vi "Main.vi"() -> ()   [LabVIEW 2019]
uses:
  Control Timer.ctl
  <vilib>/vision/Image Controls.llb/IMAQ Image.ctl
  <vilib>/Utility/file.llb/Read Delimited Spreadsheet (string).vi
panel:
  out "Camera Feed":T1(plugin-control)
  in  "Empty Spot":bool
  in  "Spot Number":i8(knob)=1 scale=1.0..6.0
  in  "SnapPhoto":bool
  in  "Tab Control":T2(tab)
  out "Parking Spot #6":T3
  out "Time of Arrival 6":timestamp
  out "Ticket Expiration Time 6":timestamp
  out "Ticket Validation\n          Status 6":bool
  out "Ticket Length\n(Seconds) 6":dbl
  out "Time left\n(Seconds) 6":dbl
  out "Parking Spot #5":T3
  out "Time left\n(Seconds) 5":dbl
  out "Ticket Validation\n          Status 5":bool
  out "Time of Arrival 5":timestamp
  out "Ticket Expiration Time 5":timestamp
  out "Ticket Length\n(Seconds) 5":dbl
  out "Parking Spot #4":T3
  out "Time left\n(Seconds) 4":dbl
  out "Time of Arrival 4":timestamp
  out "Ticket Validation\n          Status 4":bool
  out "Ticket Expiration Time 4":timestamp
  out "Ticket Length\n(Seconds) 4":dbl
  out "Parking Spot #3 (Reserved for Handicapped people)":T3
  out "Ticket Validation\n          Status 3":bool
  out "Ticket Expiration Time 3":timestamp
  out "Time of Arrival 3":timestamp
  out "Ticket Length\n(Seconds) 3":dbl
  out "Time left\n(Seconds) 3":dbl
  out "Parking Spot #2":T3
  out "Time left\n(Seconds) 2":dbl
  out "Time of Arrival 2":timestamp
  out "Ticket Validation\n          Status 2":bool
  out "Ticket Expiration Time 2":timestamp
  out "Ticket Length\n(Seconds) 2":dbl
  out "Ticket Expiration Time":timestamp
  out "Time of Arrival":timestamp
  out "Ticket Validation\n          Status":bool
  out "Parking Spot #1":T3
  out "Time left\n(Seconds)":dbl
  out "Ticket Length\n(Seconds)":dbl
  in  "UseCamera":bool
  out "Error Terminal Out":errorcluster
  in  "Licence Database filepath":path=path "C:/Users/nedel/Desktop/PSR 'Veljko' Mk.Ia/Files/Databases/LicenceDatabase.csv"
  out "error out 6":errorcluster
  out "error out 5":errorcluster
  out "error out":errorcluster
  out "error out 4":errorcluster
  out "error out 2":errorcluster
  out "error out 3":errorcluster
  in  "Ticket Database filepath":path=path "C:/Users/nedel/Desktop/PSR 'Veljko' Mk.Ia/Files/Databases/TicketDatabase.csv"
  in  "Criminal record database":path=path "C:/Users/nedel/Desktop/PSR 'Veljko' Mk.Ia/Files/Databases/CriminalRecordsDatabase.csv"
  in  "Python program filepath":path=path "C:/Users/nedel/Desktop/PSR 'Veljko' Mk.Ia/Python/gopro.py"
  in  "Handicapped Right Database":path=path "C:/Users/nedel/Desktop/PSR 'Veljko' Mk.Ia/Files/Databases/HandicappedRightDatabase.csv"
  in  "ImageFilepath":path=path "C:/Users/nedel/Desktop/PSR 'Veljko' Mk.Ia/Python/gopro.py"
  in  "stop":bool
  # "SCADA controls"
  # "Image acquisition might take some time\ndue to hardware limitations\n(Approximately 10 seconds)"
  # "!"
  # "6"
  # "5"
  # "4"
  # "3"
  # "2"
  # "1"
  # "UseFile"
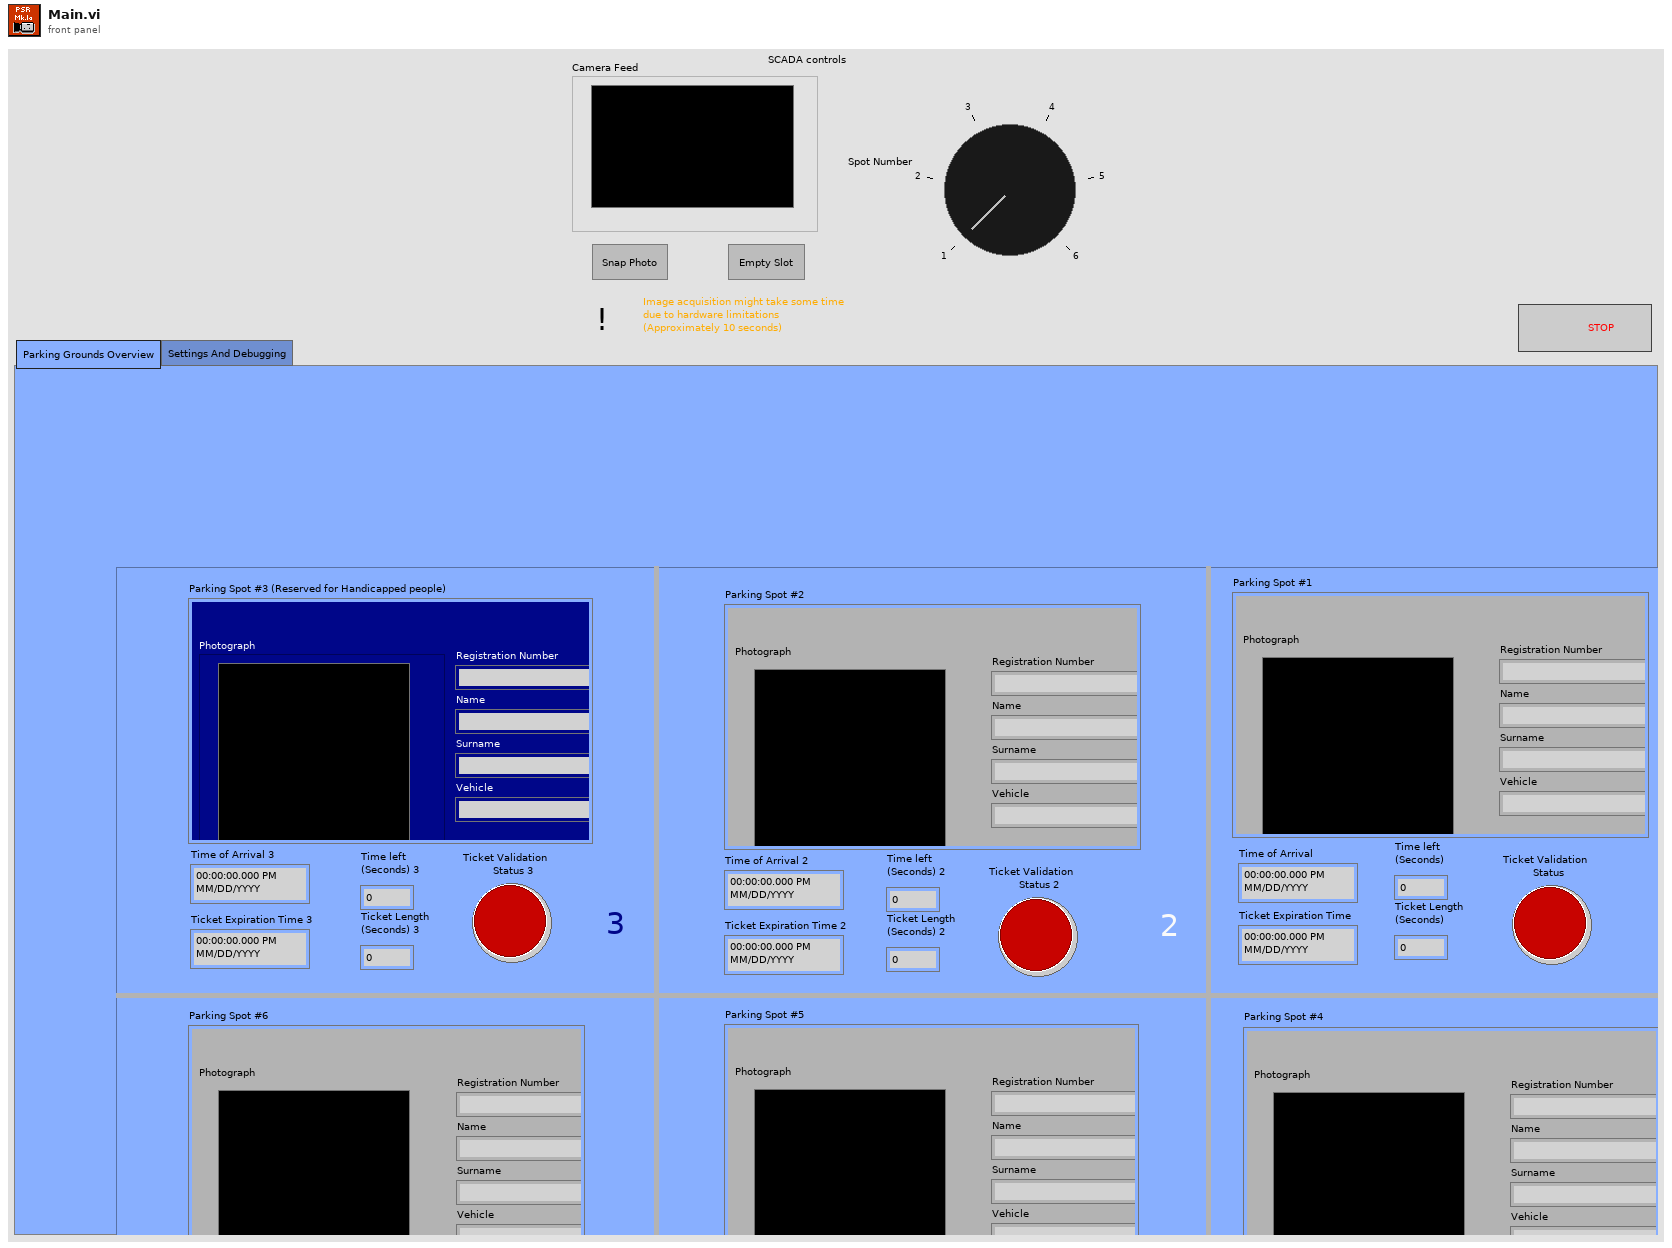
[diagram p1: front panel]
types:
  T1 = typedef "IMAQ Image.ctl" = refnum<image>
  T2 = enum32{"Parking Grounds Overview", "Settings And Debugging"}
  T3 = cluster{"Registration Number":string, "Name":string, "Surname":string, "Vehicle":string, "Photograph":T1}
  T4 = cluster{"Registration Number":string, "Name":string, "Surname":string, "Place":string, "Photograph":T1}
  T5 = typedef "Control Timer.ctl" = enum16{"Timecheck", "Reset"}
  T6 = typedef "Image Type" = u32
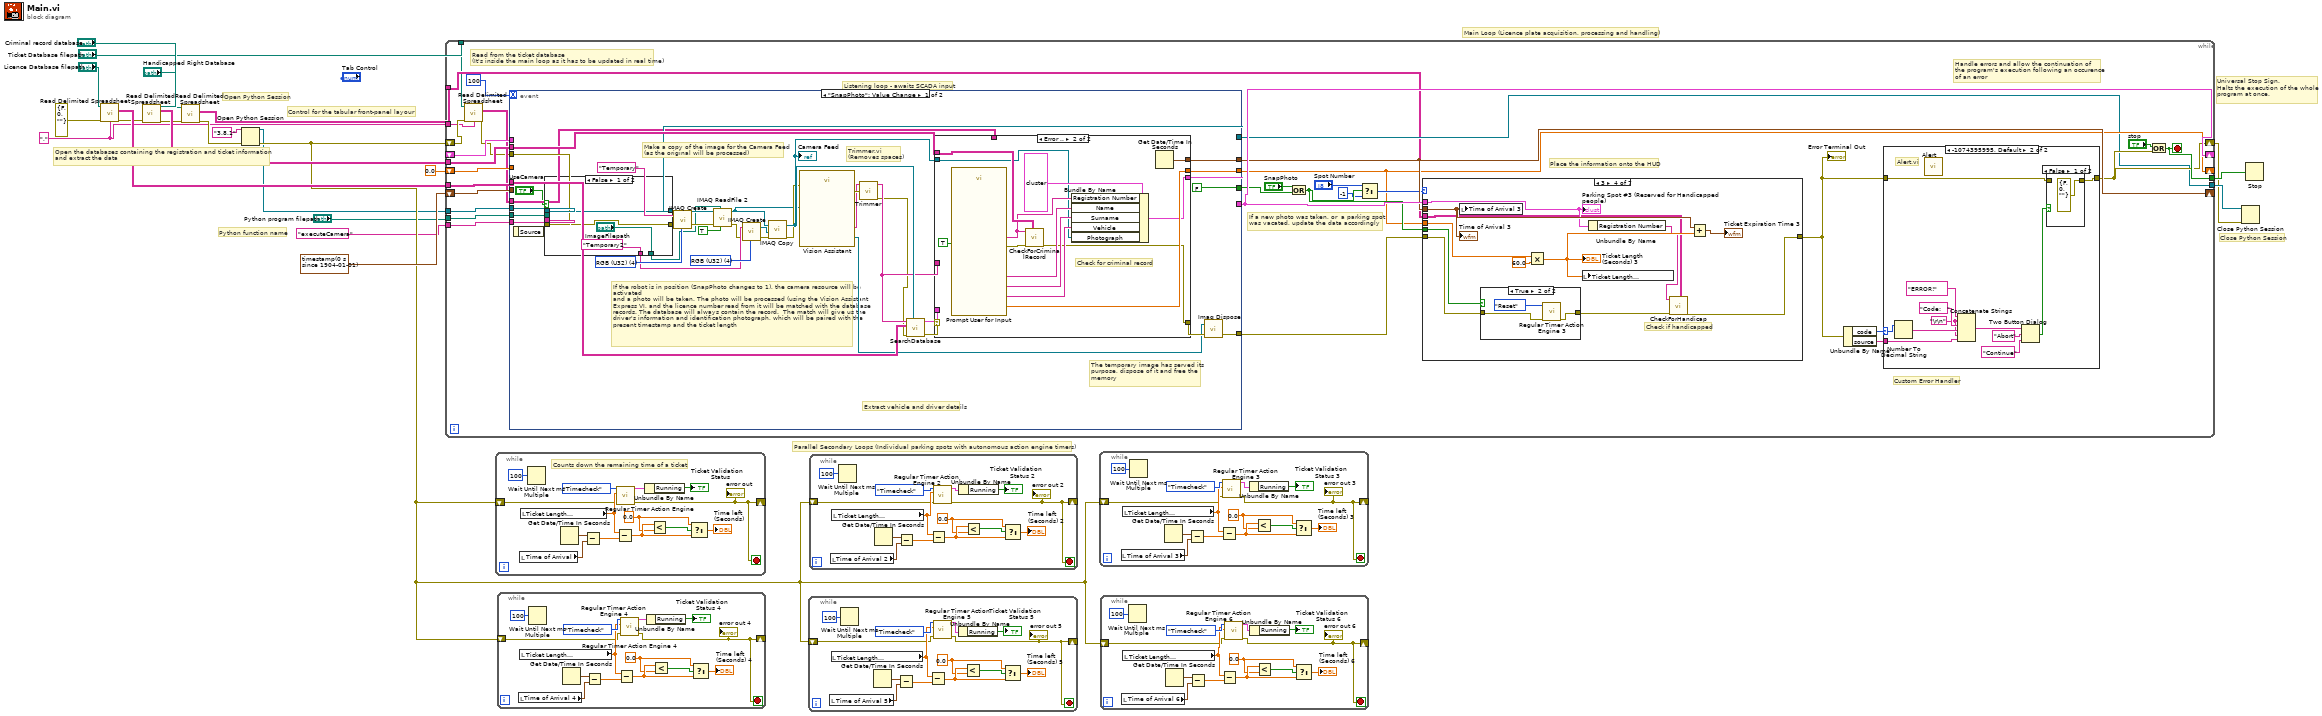
[diagram p0: block diagram]
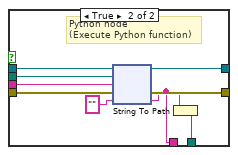
[diagram p2: hidden frame]
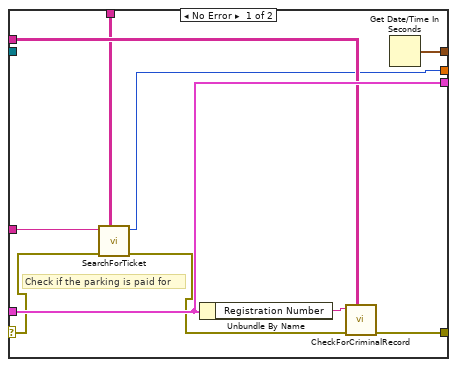
[diagram p3: hidden frame]
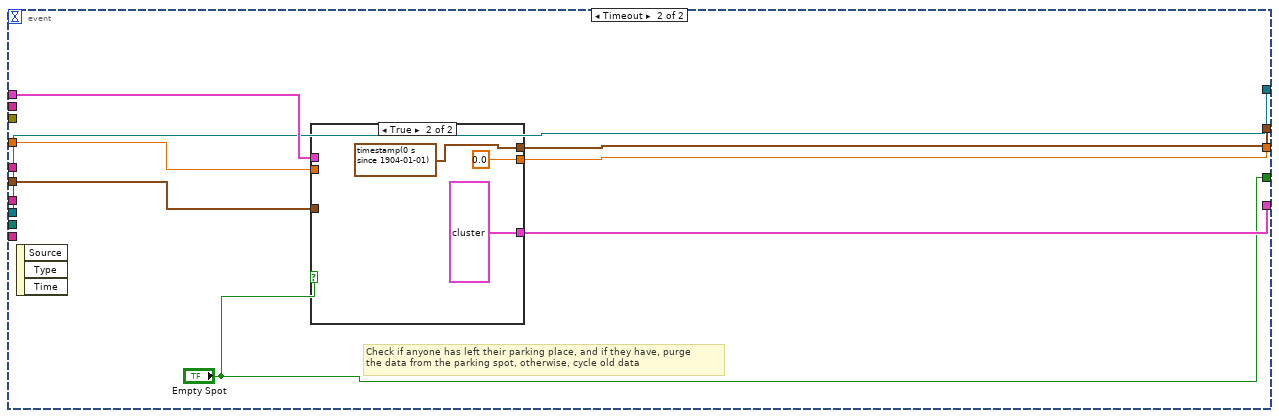
[diagram p4: hidden frame]
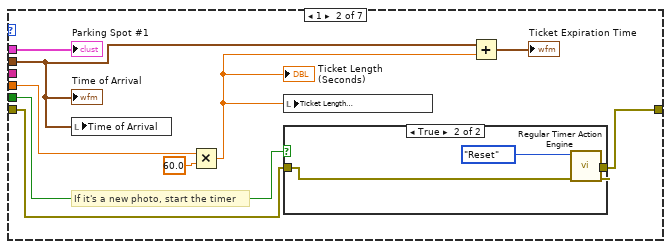
[diagram p7: hidden frame]
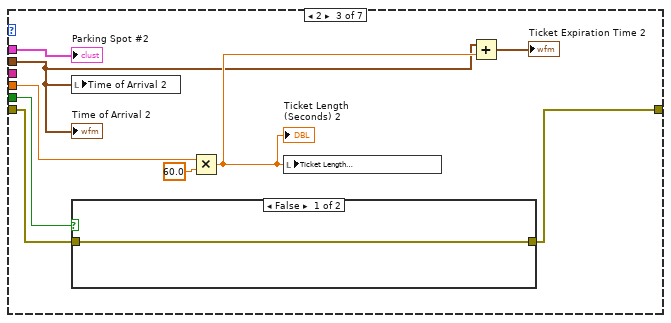
[diagram p9: hidden frame]
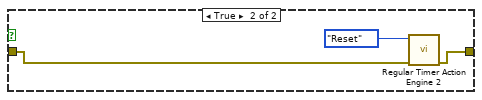
[diagram p10: hidden frame]
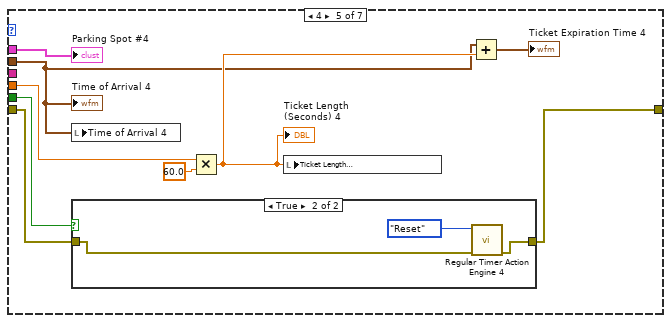
[diagram p12: hidden frame]
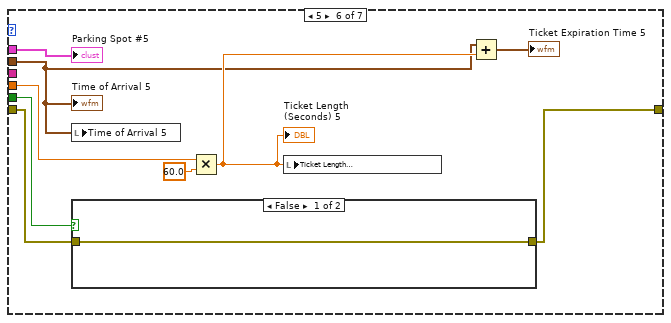
[diagram p14: hidden frame]
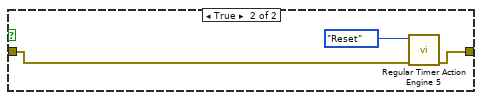
[diagram p15: hidden frame]
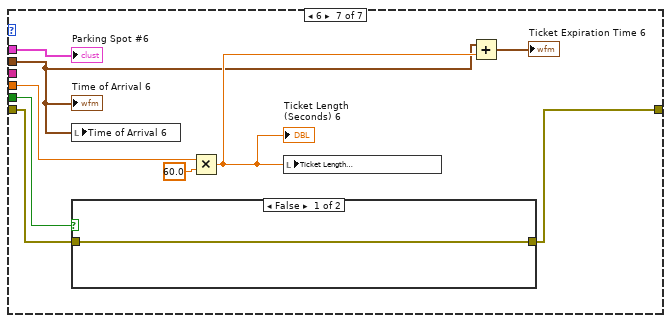
[diagram p16: hidden frame]
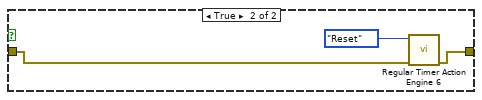
[diagram p17: hidden frame]
diagram:
  w1 = "," ("delimiter (\\t)")
  # "Open Python Session"
  # "Close Python Session"
  # "Python function name"
  # "Control for the tabular front-panel layour"
  # "Parallel Secondary Loops (Individual parking spots with autonomous action engine timers)"
  # "Main Loop (Licence plate acquisition, processing and handling)"
  # "Universal Stop Sign.\nHalts the execution of the whole\nprogram at once."
  # "Open the databases containing the registration and ticket information\nand extract the data"
  n1 = call-poly <vilib>:"Read Delimited Spreadsheet.vi"("file path (dialog if empty)"="Licence Database filepath", "error in (no error)"=errorcluster {"status"=FALSE, "code"=0, "source"=""} ("error in"), "delimiter (\\t)"=w1) -> ("all rows"=w22:string[][], "error out"=w3:errorcluster)  [unwired: 7 in, 4 out]
  n2 = call-poly <vilib>:"Read Delimited Spreadsheet.vi"("file path (dialog if empty)"="Criminal record database", "error in (no error)"=w3) -> ("all rows"=w16:string[][], "error out"=w6:errorcluster)  [unwired: 8 in, 4 out]
  n3 = call-poly <vilib>:"Read Delimited Spreadsheet.vi"("file path (dialog if empty)"="Handicapped Right Database", "error in (no error)"=w6) -> ("all rows"=w4:string[][], "error out"=w5:errorcluster)  [unwired: 8 in, 4 out]
  n4 = Open Python Session(python version="3.8.1" ("Python version"), 3:w5) -> (session out=w13:refnum<k35>, error out=w14:errorcluster)  [unwired: 1 in]
  n5 = while {
    shift-right: [w38] -> w8
    shift-left: w14 -> [w25]
    tunnel: w22 -> [w53]
    tunnel: [w51] -> w9
    shift-right: [w46] -> _
    shift-left: _ -> [w47]
    shift-right: [w37] -> _
    shift-left: 0.0 ("Ticket Length\n(Minutes)") -> [w48]
    shift-right: [w45] -> _
    shift-left: timestamp(0 s since 1904-01-01) ("seconds since 1Jan1904") -> [w49]
    tunnel: w16 -> [w36]
    tunnel: w13 -> [w34]
    tunnel: "Python program filepath" -> [w33]
    tunnel: "executeCamera" ("function name") -> [w32]
    tunnel: [w31] -> w10
    tunnel: w4 -> [w30]
    tunnel: "Ticket Database filepath" -> [w27]
    tunnel: w1 -> [w23]
    stop <- w51 stop-if-true
    # "Read from the ticket database\n(It's inside the main loop as it has to be updated in real time)"
    # "Place the information onto the HUD"
    # "Listening loop - awaits SCADA input"
    # "Custom Error Handler"
    # "Handle errors and allow the continuation of \nthe program's execution following an occurence\nof an error"
    # "If a new photo was taken, or  a parking spot\nwas vacated, update the data accordingly"
    n6 = call-poly <vilib>:"Read Delimited Spreadsheet.vi"("file path (dialog if empty)"=w27, "error in (no error)"=w25, "delimiter (\\t)"=w23) -> ("all rows"=w26:string[][], "error out"=w24:errorcluster)  [unwired: 7 in, 4 out]
    n7 = event shown="[0] \"SnapPhoto\": Value Change" {
      selector: _ -> [_ _]
      dyn-events: _ -> [_ _]
      timeout: 100 -> [_ _]
      tunnel: w53 -> [w82 _]
      tunnel: [w83 w135] -> w46
      tunnel: [w77 _] -> w50
      tunnel: [w80 w134] -> w37
      tunnel: [w81 w133] -> w45
      tunnel: [FALSE ("Empty Spot") "Empty Spot"] -> w28
      tunnel: w49 -> [_ w131]
      tunnel: w48 -> [_ w130]
      tunnel: w47 -> [_ w129]
      tunnel: w26 -> [w58 _]
      tunnel: w36 -> [w79 _]
      tunnel: w34 -> [w76 w128]
      tunnel: w33 -> [w75 _]
      tunnel: w32 -> [w74 _]
      tunnel: w24 -> [w73 _]
      tunnel: [w71 w128] -> w31
      event "SnapPhoto": Value Change {
        w70 = T6 4 items=["Grayscale (U8)", "Grayscale (I16)", "Grayscale (SGL)", "Complex (CSG)", "RGB (U32)", "HSL (U32)", "RGB (U64)", "Grayscale (U16)"] ("Image Type")
        w86 = T6 4 items=["Grayscale (U8)", "Grayscale (I16)", "Grayscale (SGL)", "Complex (CSG)", "RGB (U32)", "HSL (U32)", "RGB (U64)", "Grayscale (U16)"] ("Image Type")
        # "Trimmer.vi\n(Removes spaces)"
        # "Extract vehicle and driver details"
        # "Make a copy of the image for the Camera Feed\n(as the original will be processed)"
        # "The temporary image has served its\npurpose, dispose of it and free the\nmemory"
        # "If the robot is in position (SnapPhoto changes to 1), the camera resource will be activated\nand a photo will be taken. The photo will be processed (using the Vision Assistant Express VI, and the licence number read from it will be matched with the database records. The database will always contain the record.  The match will give us the driver's information and identification photograph, which will be paired with the present timestamp and the ticket length"
        n8 = event-data() -> ()  [unwired: 1 in, 1 out]
        n9 = case shown="False" "UseCamera" {
          tunnel: w76 -> [w95 w104]
          tunnel: w75 -> [_ w103]
          tunnel: w74 -> [_ w102]
          tunnel: w73 -> [w92 w101]
          tunnel: [w92 w100] -> w72
          tunnel: [w95 w99] -> w71
          tunnel: ["Temporary2" w97] -> w67
          tunnel: ["ImageFilepath" w96] -> w56
          frame False {
          }
          frame True {
            # "Python node\n(Execute Python function)"
            n10 = node(w104, w103, w102, w101, "") -> (w99:refnum<k35>, w100:errorcluster, w97:string)  [unwired: 2 out]
            n11 = String To Path(string=w97) -> (path=w96:path)
          }
        }
        n12 = call "IMAQ Create"("Image Name"="Temporary", "Image Type"=w86, "error in (no error)"=w72) -> ("New Image"=w89:T1, "error out"=w88:errorcluster)  [unwired: 2 in]
        n13 = call "IMAQ ReadFile 2"("Use File Path Image Type"=TRUE, "File Path"=w56, "error in (no error)"=w88, "Image"=w89) -> ("error out"=w66:errorcluster, "Image Out"=w63:T1)  [unwired: 3 in, 3 out]
        n14 = call "IMAQ Create"("Image Name"=w67, "Image Type"=w70, "error in (no error)"=w66) -> ("New Image"=w68:T1, "error out"=w69:errorcluster)  [unwired: 2 in]
        n15 = call "IMAQ Copy"("error in (no error)"=w69, "Image Dst"=w68, "Image Src"=w63) -> ("error out"=w64:errorcluster, "Image Dst Out"=w65:T1)  [unwired: 3 in]
        "Camera Feed" <- w65
        n16 = call "Vision Assistant"("Image In"=w63, "error in"=w64) -> ("Image Out"=w61:T1, "String (OCR/OCV)"=w60:string, "error out"=w62:errorcluster)  [unwired: 23 in]
        n17 = call "Trimmer.vi"("error in"=w62, "String In"=w60) -> ("error out"=w57:errorcluster, "result string"=w59:string)  [unwired: 8 in]
        n18 = call "SearchDatabase.vi"("Licence"=w59, "Image in"=w65, "Database"=w82, "error in"=w57) -> ("Individual"=w84:T4, "error out"=w85:errorcluster)  [unwired: 3 in]
        n19 = case shown="Error .." w85 {
          selector: w85 -> [w106 _]
          tunnel: [w113 w119] -> w78
          tunnel: [w112 w120] -> w83
          tunnel: w84 -> [w112 _]
          tunnel: [w107 w122] -> w80
          tunnel: [w114 w121] -> w81
          tunnel: w79 -> [w110 w118]
          tunnel: w65 -> [_ w115]
          tunnel: w59 -> [w109 _]
          tunnel: w58 -> [w108 _]
          frame No Error {
            # "Check if the parking is paid for"
            n20 = call "SearchForTicket.vi"("Licence"=w109, "error in"=w106, "Database"=w108) -> ("TicketDuration"=w107:i32, "error out"=w105:errorcluster)  [unwired: 6 in]
            n21 = Unbundle By Name(w112) -> ("Registration Number"=w111:string)
            n22 = call "CheckForCriminalRecord.vi"("Licence"=w111, "error in"=w105, "Database"=w110) -> ("error out"=w113:errorcluster)  [unwired: 7 in]
            n23 = Get Date/Time In Seconds() -> (seconds since 1Jan1904=w114:timestamp)
          }
          frame Error {
            # "Check for criminal record"
            n24 = call "Prompt User for Input"("Enable"=TRUE) -> ("Ticked duration (minutes)"=w122:dbl, "Vehicle"=w123:string, "Surname"=w124:string, "Name"=w125:string, "Registration number"=w117:string, "error out"=w116:errorcluster)  [unwired: 12 in, 1 out]
            n25 = call "CheckForCriminalRecord.vi"("Licence"=w117, "error in"=w116, "Database"=w118) -> ("error out"=w119:errorcluster)  [unwired: 7 in]
            n26 = Bundle By Name(cluster=T3 {"Registration Number"="", "Name"="", "Surname"="", "Vehicle"="", "Photograph"=refnum} ("Individual"), "Registration Number"=w117, "Name"=w125, "Surname"=w124, "Vehicle"=w123, "Photograph"=w115) -> (w120:T3)
            n27 = Get Date/Time In Seconds() -> (seconds since 1Jan1904=w121:timestamp)
          }
        }
        n28 = call "Imaq Dispose"("Image"=w61, "error in (no error)"=w78) -> ("error out"=w77:errorcluster)  [unwired: 4 in]
      }
      event Timeout {
        # "Check if anyone has left their parking place, and if they have, purge \nthe data from the parking spot, otherwise, cycle old data"
        n29 = event-data() -> ()  [unwired: 1 in, 3 out]
        n30 = case shown="True" "Empty Spot" {
          tunnel: [w136 T4 {"Registration Number"="", "Name"="", "Surname"="", "Place"="", "Photograph"=refnum} ("Individual")] -> w135
          tunnel: [w137 0.0 ("Ticket Length\n(Minutes)")] -> w134
          tunnel: [w138 timestamp(0 s since 1904-01-01) ("seconds since 1Jan1904")] -> w133
          tunnel: w131 -> [w138 _]
          tunnel: w130 -> [w137 _]
          tunnel: w129 -> [w136 _]
          frame False {
          }
          frame True {
          }
        }
      }
    }
    n31 = Or(x="SnapPhoto", y=w28) -> (x .or. y?=w44:bool)
    n32 = Select(t="Spot Number", s=w44, f=i8 -1) -> (s? t:f=w41:i8)
    n33 = case shown="3" w41 {
      tunnel: w46 -> [_ w151 w164 w171 w193 w206 w219]
      tunnel: w50 -> [w142 w150 w159 w176 w187 w201 w214]
      tunnel: w37 -> [_ w146 w160 w177 w189 w202 w215]
      tunnel: [w142 w149 w158 w173 w188 w200 w213] -> w39
      tunnel: w45 -> [_ w143 w156 w174 w186 w198 w211]
      tunnel: w44 -> [_ w144 w157 w175 w185 w199 w212]
      tunnel: w30 -> [_ _ _ w169 _ _ _]
      frame -1, Default {
      }
      frame 1 {
        # "If it's a new photo, start the timer"
        n34 = local write "Time of Arrival"(w143) -> ()
        n35 = Multiply(x=w146, y=60.0) -> (x*y=w145:dbl)
        "Ticket Length\n(Seconds)" <- w145
        n36 = local write "Ticket Length\n(Seconds)"(w145) -> ()
        n37 = case shown="True" w144 {
          tunnel: w150 -> [w152 w155]
          tunnel: [w152 w153] -> w149
          frame False {
          }
          frame True {
            n38 = call "Regular Timer Action Engine.vi"("Enum"=Control_Timer."Reset", "error in"=w155) -> ("error out"=w153:errorcluster)  [unwired: 7 in, 1 out]
          }
        }
        n39 = Add(x=w143, y=w145) -> (x+y=→"Ticket Expiration Time":timestamp)
        "Parking Spot #1" <- w151
        "Time of Arrival" <- w143
      }
      frame 2 {
        n40 = local write "Time of Arrival 2"(w156) -> ()
        n41 = case shown="False" w157 {
          tunnel: w159 -> [w165 w167]
          tunnel: [w165 w166] -> w158
          frame False {
          }
          frame True {
            n42 = call "Regular Timer Action Engine 2.vi"("Enum"=Control_Timer."Reset", "error in"=w167) -> ("error out"=w166:errorcluster)  [unwired: 7 in, 1 out]
          }
        }
        n43 = Multiply(x=w160, y=60.0) -> (x*y=w161:dbl)
        "Ticket Length\n(Seconds) 2" <- w161
        n44 = local write "Ticket Length\n(Seconds) 2"(w161) -> ()
        n45 = Add(x=w156, y=w161) -> (x+y=→"Ticket Expiration Time 2":timestamp)
        "Parking Spot #2" <- w164
        "Time of Arrival 2" <- w156
      }
      frame 3 {
        # "Check if handicapped"
        n46 = local write "Time of Arrival 3"(w174) -> ()
        n47 = case shown="True" w175 {
          tunnel: w176 -> [w181 w183]
          tunnel: [w181 w182] -> w172
          frame False {
          }
          frame True {
            n48 = call "Regular Timer Action Engine 3.vi"("Enum"=Control_Timer."Reset", "error in"=w183) -> ("error out"=w182:errorcluster)  [unwired: 7 in, 1 out]
          }
        }
        n49 = Multiply(x=w177, y=60.0) -> (x*y=w178:dbl)
        "Ticket Length\n(Seconds) 3" <- w178
        n50 = local write "Ticket Length\n(Seconds) 3"(w178) -> ()
        n51 = Unbundle By Name(w171) -> ("Registration Number"=w170:string)
        n52 = call "CheckForHandicap.vi"("Licence"=w170, "error in"=w172, "Database"=w169) -> ("error out"=w173:errorcluster)  [unwired: 7 in]
        n53 = Add(x=w174, y=w178) -> (x+y=→"Ticket Expiration Time 3":timestamp)
        "Parking Spot #3 (Reserved for Handicapped people)" <- w171
        "Time of Arrival 3" <- w174
      }
      frame 4 {
        n54 = local write "Time of Arrival 4"(w186) -> ()
        n55 = case shown="True" w185 {
          tunnel: [w194 w197] -> w188
          tunnel: w187 -> [w194 w196]
          frame False {
          }
          frame True {
            n56 = call "Regular Timer Action Engine 4.vi"("Enum"=Control_Timer."Reset", "error in"=w196) -> ("error out"=w197:errorcluster)  [unwired: 7 in, 1 out]
          }
        }
        n57 = Multiply(x=w189, y=60.0) -> (x*y=w192:dbl)
        "Ticket Length\n(Seconds) 4" <- w192
        n58 = local write "Ticket Length\n(Seconds) 4"(w192) -> ()
        n59 = Add(x=w186, y=w192) -> (x+y=→"Ticket Expiration Time 4":timestamp)
        "Parking Spot #4" <- w193
        "Time of Arrival 4" <- w186
      }
      frame 5 {
        n60 = local write "Time of Arrival 5"(w198) -> ()
        n61 = case shown="False" w199 {
          tunnel: w201 -> [w207 w209]
          tunnel: [w207 w208] -> w200
          frame False {
          }
          frame True {
            n62 = call "Regular Timer Action Engine 5.vi"("Enum"=Control_Timer."Reset", "error in"=w209) -> ("error out"=w208:errorcluster)  [unwired: 7 in, 1 out]
          }
        }
        n63 = Multiply(x=w202, y=60.0) -> (x*y=w203:dbl)
        "Ticket Length\n(Seconds) 5" <- w203
        n64 = local write "Ticket Length\n(Seconds) 5"(w203) -> ()
        n65 = Add(x=w198, y=w203) -> (x+y=→"Ticket Expiration Time 5":timestamp)
        "Parking Spot #5" <- w206
        "Time of Arrival 5" <- w198
      }
      frame 6 {
        n66 = local write "Time of Arrival 6"(w211) -> ()
        n67 = case shown="False" w212 {
          tunnel: w214 -> [w220 w223]
          tunnel: [w220 w221] -> w213
          frame False {
          }
          frame True {
            n68 = call "Regular Timer Action Engine 6.vi"("Enum"=Control_Timer."Reset", "error in"=w223) -> ("error out"=w221:errorcluster)  [unwired: 7 in, 1 out]
          }
        }
        n69 = Multiply(x=w215, y=60.0) -> (x*y=w218:dbl)
        "Ticket Length\n(Seconds) 6" <- w218
        n70 = local write "Ticket Length\n(Seconds) 6"(w218) -> ()
        n71 = Add(x=w211, y=w218) -> (x+y=→"Ticket Expiration Time 6":timestamp)
        "Parking Spot #6" <- w219
        "Time of Arrival 6" <- w211
      }
    }
    "Error Terminal Out" <- w39
    n72 = Unbundle By Name(w39) -> ("code"=w40:i32, "source"=w35:string)
    n73 = case shown="-1074395995, Default" w40 {
      selector: w40 -> [_ w231]
      tunnel: [w224 w233] -> w38
      tunnel: w39 -> [w224 w229]
      tunnel: w35 -> [_ w225]
      frame 0 {
      }
      frame -1074395995, Default {
        w226 = "\r\n"
        # "Alert.vi"
        n74 = Number To Decimal String(number=w231) -> (decimal integer string=w227:string)  [unwired: 1 in]
        n75 = call "Alert.vi"() -> ()  [unwired: 12 in]
        n76 = Concatenate Strings("ERROR!" ("message"), w226, "Code:   " ("string"), w227, w226, w225) -> (w230:string)
        n77 = Two Button Dialog(message=w230, 1:"Continue" ("F button name (\"Cancel\")"), 2:"Abort" ("T button name (\"OK\")")) -> (T button?=w236:bool)
        n78 = case shown="False" w236 {
          tunnel: [errorcluster {"status"=FALSE, "code"=0, "source"=""} ("error out") w238] -> w233
          tunnel: w229 -> [_ w238]
          frame False {
          }
          frame True {
          }
        }
      }
    }
    n79 = Or(x="stop", y=w38) -> (x .or. y?=w51:bool)
  }
  n80 = while {
    shift-right: [w239] -> _
    shift-left: w14 -> [w240]
    stop <- w239 stop-if-true
    w242 = 0.0 ("y")
    # "Counts down the remaining time of a ticket"
    n81 = local read "Time of Arrival"() -> (w248:timestamp)
    n82 = local read "Ticket Length\n(Seconds)"() -> (w247:dbl)
    n83 = Wait Until Next ms Multiple(millisecond multiple=u32 100 ("milliseconds to wait")) -> ()  [unwired: 1 out]
    n84 = Get Date/Time In Seconds() -> (seconds since 1Jan1904=w249:timestamp)
    n85 = Subtract(x=w249, y=w248) -> (x-y=w246:dbl)
    n86 = Subtract(x=w247, y=w246) -> (x-y=w243:dbl)
    n87 = call "Regular Timer Action Engine.vi"("Enum"=Control_Timer."Timecheck", "Time Target"=w247, "error in"=w240) -> ("Status"=w251:cluster{"Running":bool, "Done":bool}, "error out"=w239:errorcluster)  [unwired: 6 in]
    "error out" <- w239
    n88 = Unbundle By Name(w251) -> ("Running"=→"Ticket Validation\n          Status":bool)
    n89 = Less?(x=w243, y=w242) -> (x < y?=w244:bool)
    n90 = Select(t=w242, s=w244, f=w243) -> (s? t:f=→"Time left\n(Seconds)":dbl)
  }
  n91 = while {
    shift-right: [w253] -> _
    shift-left: w14 -> [w254]
    stop <- w253 stop-if-true
    w259 = 0.0 ("y")
    n92 = local read "Time of Arrival 4"() -> (w264:timestamp)
    n93 = local read "Ticket Length\n(Seconds) 4"() -> (w255:dbl)
    n94 = Wait Until Next ms Multiple(millisecond multiple=u32 100 ("milliseconds to wait")) -> ()  [unwired: 1 out]
    n95 = Get Date/Time In Seconds() -> (seconds since 1Jan1904=w265:timestamp)
    n96 = Subtract(x=w265, y=w264) -> (x-y=w263:dbl)
    n97 = Subtract(x=w255, y=w263) -> (x-y=w260:dbl)
    n98 = call "Regular Timer Action Engine 4.vi"("Enum"=Control_Timer."Timecheck", "Time Target"=w255, "error in"=w254) -> ("Status"=w258:cluster{"Running":bool, "Done":bool}, "error out"=w253:errorcluster)  [unwired: 6 in]
    "error out 4" <- w253
    n99 = call "Regular Timer Action Engine 4.vi"() -> ()  [unwired: 9 in, 2 out]
    n100 = Unbundle By Name(w258) -> ("Running"=→"Ticket Validation\n          Status 4":bool)
    n101 = Less?(x=w260, y=w259) -> (x < y?=w261:bool)
    n102 = Select(t=w259, s=w261, f=w260) -> (s? t:f=→"Time left\n(Seconds) 4":dbl)
  }
  n103 = while {
    shift-right: [w267] -> _
    shift-left: w14 -> [w268]
    stop <- w267 stop-if-true
    w273 = 0.0 ("y")
    n104 = local read "Time of Arrival 5"() -> (w278:timestamp)
    n105 = local read "Ticket Length\n(Seconds) 5"() -> (w269:dbl)
    n106 = Wait Until Next ms Multiple(millisecond multiple=u32 100 ("milliseconds to wait")) -> ()  [unwired: 1 out]
    n107 = Get Date/Time In Seconds() -> (seconds since 1Jan1904=w279:timestamp)
    n108 = Subtract(x=w279, y=w278) -> (x-y=w277:dbl)
    n109 = Subtract(x=w269, y=w277) -> (x-y=w274:dbl)
    n110 = call "Regular Timer Action Engine 5.vi"("Enum"=Control_Timer."Timecheck", "Time Target"=w269, "error in"=w268) -> ("Status"=w272:cluster{"Running":bool, "Done":bool}, "error out"=w267:errorcluster)  [unwired: 6 in]
    "error out 5" <- w267
    n111 = Unbundle By Name(w272) -> ("Running"=→"Ticket Validation\n          Status 5":bool)
    n112 = Less?(x=w274, y=w273) -> (x < y?=w275:bool)
    n113 = Select(t=w273, s=w275, f=w274) -> (s? t:f=→"Time left\n(Seconds) 5":dbl)
  }
  n114 = while {
    shift-right: [w281] -> _
    shift-left: w14 -> [w282]
    stop <- w281 stop-if-true
    w287 = 0.0 ("y")
    n115 = local read "Time of Arrival 2"() -> (w292:timestamp)
    n116 = local read "Ticket Length\n(Seconds) 2"() -> (w283:dbl)
    n117 = Wait Until Next ms Multiple(millisecond multiple=u32 100 ("milliseconds to wait")) -> ()  [unwired: 1 out]
    n118 = Get Date/Time In Seconds() -> (seconds since 1Jan1904=w293:timestamp)
    n119 = Subtract(x=w293, y=w292) -> (x-y=w291:dbl)
    n120 = Subtract(x=w283, y=w291) -> (x-y=w288:dbl)
    n121 = call "Regular Timer Action Engine 2.vi"("Enum"=Control_Timer."Timecheck", "Time Target"=w283, "error in"=w282) -> ("Status"=w285:cluster{"Running":bool, "Done":bool}, "error out"=w281:errorcluster)  [unwired: 6 in]
    "error out 2" <- w281
    n122 = Unbundle By Name(w285) -> ("Running"=→"Ticket Validation\n          Status 2":bool)
    n123 = Less?(x=w288, y=w287) -> (x < y?=w289:bool)
    n124 = Select(t=w287, s=w289, f=w288) -> (s? t:f=→"Time left\n(Seconds) 2":dbl)
  }
  n125 = while {
    shift-right: [w295] -> _
    shift-left: w14 -> [w296]
    stop <- w295 stop-if-true
    w301 = 0.0 ("y")
    n126 = local read "Time of Arrival 3"() -> (w306:timestamp)
    n127 = local read "Ticket Length\n(Seconds) 3"() -> (w297:dbl)
    n128 = Wait Until Next ms Multiple(millisecond multiple=u32 100 ("milliseconds to wait")) -> ()  [unwired: 1 out]
    n129 = Get Date/Time In Seconds() -> (seconds since 1Jan1904=w307:timestamp)
    n130 = Subtract(x=w307, y=w306) -> (x-y=w305:dbl)
    n131 = Subtract(x=w297, y=w305) -> (x-y=w302:dbl)
    n132 = call "Regular Timer Action Engine 3.vi"("Enum"=Control_Timer."Timecheck", "Time Target"=w297, "error in"=w296) -> ("Status"=w299:cluster{"Running":bool, "Done":bool}, "error out"=w295:errorcluster)  [unwired: 6 in]
    "error out 3" <- w295
    n133 = Unbundle By Name(w299) -> ("Running"=→"Ticket Validation\n          Status 3":bool)
    n134 = Less?(x=w302, y=w301) -> (x < y?=w303:bool)
    n135 = Select(t=w301, s=w303, f=w302) -> (s? t:f=→"Time left\n(Seconds) 3":dbl)
  }
  n136 = while {
    shift-right: [w309] -> _
    shift-left: w14 -> [w310]
    stop <- w309 stop-if-true
    w315 = 0.0 ("y")
    n137 = local read "Time of Arrival 6"() -> (w320:timestamp)
    n138 = local read "Ticket Length\n(Seconds) 6"() -> (w311:dbl)
    n139 = Wait Until Next ms Multiple(millisecond multiple=u32 100 ("milliseconds to wait")) -> ()  [unwired: 1 out]
    n140 = Get Date/Time In Seconds() -> (seconds since 1Jan1904=w321:timestamp)
    n141 = Subtract(x=w321, y=w320) -> (x-y=w319:dbl)
    n142 = Subtract(x=w311, y=w319) -> (x-y=w316:dbl)
    n143 = call "Regular Timer Action Engine 6.vi"("Enum"=Control_Timer."Timecheck", "Time Target"=w311, "error in"=w310) -> ("Status"=w314:cluster{"Running":bool, "Done":bool}, "error out"=w309:errorcluster)  [unwired: 6 in]
    "error out 6" <- w309
    n144 = Unbundle By Name(w314) -> ("Running"=→"Ticket Validation\n          Status 6":bool)
    n145 = Less?(x=w316, y=w315) -> (x < y?=w317:bool)
    n146 = Select(t=w315, s=w317, f=w316) -> (s? t:f=→"Time left\n(Seconds) 6":dbl)
  }
  n147 = Close Python Session(session in=w10, error in=w8) -> ()  [unwired: 1 out]
  n148 = Stop(stop? (T)=w9) -> ()
